vi "Cluster Experiment.vi"() -> ()   [LabVIEW 2014]
panel:
  out "Boolean":bool
  out "Small Cluster":cluster{"Boolean 1":bool, "Slide value":dbl}
  out "Modified Cluster":T1 {"Slide" scale=0.0..10.0}
  in  "Cluster":T1 {"Slide" scale=0.0..10.0}
  out "Numeric":dbl
  in  "stop":bool
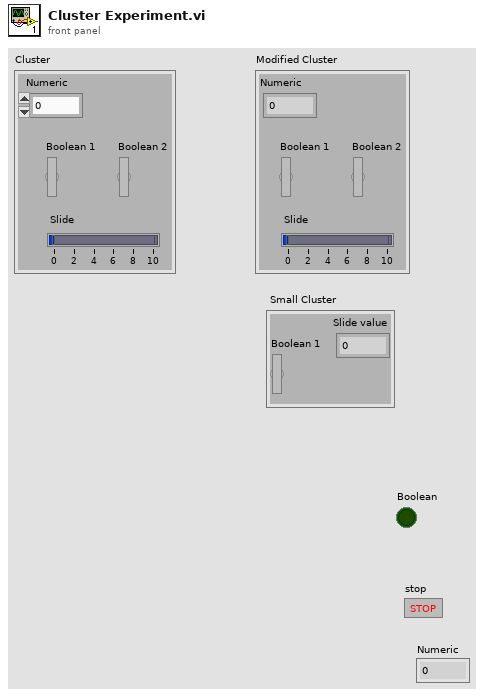
[diagram p1: front panel]
types:
  T1 = cluster{"Numeric":dbl, "Boolean 1":bool, "Boolean 2":bool, "Slide":dbl}
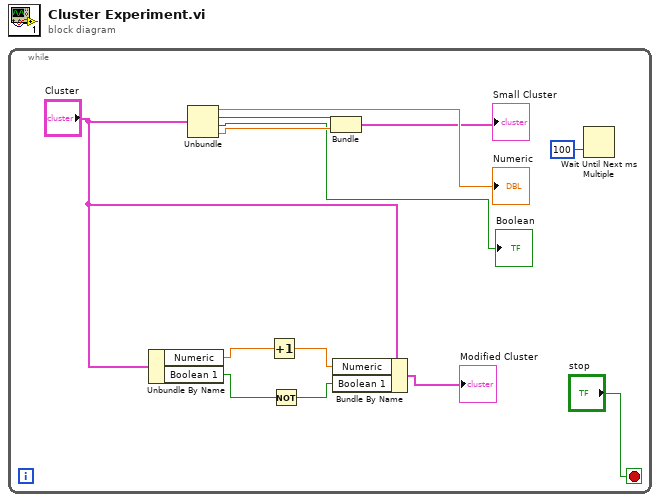
[diagram p0: block diagram]
diagram:
  n1 = while {
    stop <- "stop" stop-if-true
    n2 = Unbundle By Name("Cluster") -> ("Numeric"=w9:dbl, "Boolean 1"=w8:bool)
    n3 = Unbundle("Cluster") -> ("Numeric"=→"Numeric":dbl, "Boolean 1"=w13:bool, "Boolean 2"=→"Boolean":bool, "Slide"=w12:dbl)
    n4 = Increment(x=w9) -> (x+1=w5:dbl)
    n5 = Not(x=w8) -> (.not. x?=w6:bool)
    n6 = Bundle("Boolean 1"=w13, "Slide"=w12) -> (→"Small Cluster":cluster{"Boolean 1":bool, "Slide":dbl})  [unwired: 1 in]
    n7 = Bundle By Name(cluster="Cluster", "Numeric"=w5, "Boolean 1"=w6) -> (→"Modified Cluster":T1)
    n8 = Wait Until Next ms Multiple(millisecond multiple=u32 100) -> ()  [unwired: 1 out]
  }
